vi "find_new_direction.vi"(11 "NXT":T1={"Hardware"="NXT", "Flattened String"=""}) -> (0 "right(T)/left(F)":bool, 1 "angle":dbl, 3 "NXT 2":T1={"Hardware"="NXT", "Flattened String"=""})   [LabVIEW 2012]
uses:
  <vilib>/NXT/Subs/LVHSConnector.ctl
  <vilib>/NXT/Subs/MotorOutput.ctl
  <vilib>/NXT/Block Support/NXT_InputPort.ctl
  <vilib>/NXT/Dual Mode Library/Motors/MotorOn.vi
  <vilib>/NXT/Dual Mode Library/Motors/MotorReverse.vi
  <vilib>/NXT/Dual Mode Library/Motors/MotorBrake.vi
  <vilib>/NXT/Dual Mode Library/Display/clearDisplay.vi
  <vilib>/NXT/Dual Mode Library/Waits/Wait_Num(msec).vi
  <vilib>/NXT/Dual Mode Library/Display/drawLine.vi
  <vilib>/NXT/Dual Mode Library/Waits/Wait_Num.vi
  <vilib>/NXT/Dual Mode Library/Display/drawText.vi
  <vilib>/NXT/Dual Mode Library/Display/drawNumber.vi
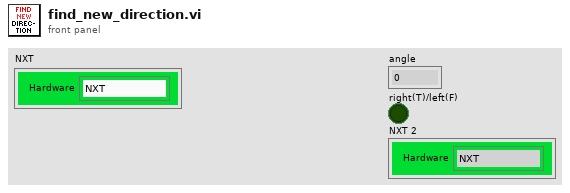
[diagram p1: front panel]
types:
  T1 = typedef "LVHSConnector.ctl" = cluster{"Hardware":string, "Flattened String":string}
  T2 = typedef "MotorOutput.ctl" = u8
  T3 = typedef "NXT_InputPort.ctl" = u8
  T4 = cluster{"x-y*floor(x/y)":i32, "Start X":i16, "x-y*floor(x/y)":i32, i16}
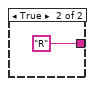
[diagram p6: hidden frame]
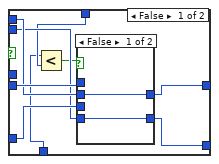
[diagram p9: hidden frame]
diagram:
  w19 = T2 5 items=["Port A"=0, "Port B"=1, "Port C"=2, "Ports A & B"=4, "Ports A & C"=5, "Ports B & C"=6, "All Ports"=3] ("Port (All Ports)")
  w25 = T2 5 items=["Port A"=0, "Port B"=1, "Port C"=2, "Ports A & B"=4, "Ports A & C"=5, "Ports B & C"=6, "All Ports"=3] ("Port (All Ports)")
  w29 = T2 2 items=["Port A"=0, "Port B"=1, "Port C"=2, "Ports A & B"=4, "Ports A & C"=5, "Ports B & C"=6, "as"=3] ("Output Port (All Ports)")
  w27 = T2 0 items=["Port A"=0, "Port B"=1, "Port C"=2, "Ports A & B"=4, "Ports A & C"=5, "Ports B & C"=6, "as"=3] ("Output Port (All Ports)")
  w43 = i16 -1 ("Start X")
  (unwired) FALSE
  w15 = TRUE
  w24 = 35 ("Power (75)")
  # "number of samples"
  # "40"
  # "rotate left"
  # "sweep sensor left"
  # "move sensor back"
  # "if sample angle is > 180, rotate right instead of left"
  # "TODO: pass array length to  find paths"
  # "TODO: pass array size to display array vi"
  # "TODO: pass array length to filter & smooth"
  # "number of distance samples"
  # "degrees"
  # "display chosen location"
  # "display list of areas"
  # "if index > 50;\n  test_index  =  100-index\n\nif current_area <  min_area:\n   if  area > current_area:\n     current_area = area\n     current_index = index\nif current_area >=  min_area:\n\n  if test_index < current_index:\n    current_area = area\n    current_index = index"
  # "morgan stanly analysist internship"
  # "minumum candedata size"
  # "find the closest turn candedate to the forward faceing direction with area over a given minimum\nor the largest if non over the minimum are found"
  # "TODO:  min distance considered, min area"
  # "msecs between distance sampling"
  # "motor power level (for scanning)"
  # "TODO:\n\n combine first and last path condidates (occuring at beginning and end of array-->should be done in the 'find paths' vi\n            \n should have minimum area, take the first one on the left(then right) side that is large enough\n\n     while current_area is less then minimum area:\n            if test_area is greator then current_area:\n                  current_area = test_area\n\ndetermindegress to turn\n\nturn, move forward until some distance is meet (?)"
  # "right max"
  # "left max"
  # "display path candedates"
  # "area"
  # "location"
  # "debug"
  # "screen: 99x63"
  n1 = call <vilib>:"ResetMotor.vi"("NXT"="NXT", "Port (All Ports)"=w25) -> ("NXT"=w26:T1)  [unwired: 2 in]
  n2 = Multiply(x=360.0 ("Max Value"), y=1.45 ("Max Value")) -> (x*y=w20:dbl)
  n3 = call-poly <vilib>:"PolyMotor.vi"("Power (75)"=w24, "NXT"=w26, "Output Port (All Ports)"=w27) -> ("NXT"=w28:T1)  [unwired: 1 in]
  n4 = call-poly <vilib>:"PolyMotor.vi"("Power (75)"=w24, "NXT"=w28, "Output Port (All Ports)"=w29) -> ("NXT"=w23:T1)  [unwired: 1 in]
  n5 = while {
    shift-right: [w78] -> w1
    shift-left: i16[] [] -> [w79]
    tunnel: [w75] -> w18
    tunnel: w15 -> [w74]
    tunnel: 7 -> [w71]
    tunnel: w23 -> [w60]
    tunnel: w20 -> [w57]
    i -> [w72]
    stop <- w58 stop-if-true
    w68 = T2 2 items=["Port A"=0, "Port B"=1, "Port C"=2, "Ports A & B"=4, "Ports A & C"=5, "Ports B & C"=6, "as"=3] ("Output Port (All Ports)")
    w69 = T2 0 items=["Port A"=0, "Port B"=1, "Port C"=2, "Ports A & B"=4, "Ports A & C"=5, "Ports B & C"=6, "as"=3] ("Output Port (All Ports)")
    w80 = T3 3 items=["Port 1", "Port 2", "Port 3", "Port 4"] ("Port (Port 4)")
    n6 = call <vilib>:"Rotation.vi"("NXT"=w60, "Port (Port A)"=w69) -> ("Angle of Rotation"=w67:i32, "NXT"=w70:T1)  [unwired: 1 in]
    n7 = Absolute Value(x=w67) -> (abs(x)=w65:i32)
    n8 = call <vilib>:"Rotation.vi"("NXT"=w70, "Port (Port A)"=w68) -> ("Angle of Rotation"=w66:i32, "NXT"=w59:T1)  [unwired: 1 in]
    n9 = Absolute Value(x=w66) -> (abs(x)=w64:i32)
    n10 = Add(x=w64, y=w65) -> (x+y=w63:i32)
    n11 = Divide(x=w63, y=2) -> (x/y=w61:dbl)
    n12 = Greater Or Equal?(x=w61, y=w57) -> (x >= y?=w58:bool)
    n13 = call <vilib>:"Sonar_cm.vi"("NXT"=w59, "Port (Port 4)"=w80) -> ("Distance (cm)"=w73:i16, "NXT"=w77:T1)  [unwired: 1 in]
    n14 = Build Array (concatenate)(w79, w73) -> (w78:i16[])
    n15 = call-poly <vilib>:"PolyWait.vi"("Time (100 msec)"=w71, "NXT"=w77) -> ("NXT"=w76:T1)  [unwired: 2 in]
    n16 = case shown="True" w74 {
      tunnel: w76 -> [w81 w91]
      tunnel: [w81 w92] -> w75
      tunnel: w73 -> [_ w90]
      tunnel: w72 -> [_ w83]
      frame False {
      }
      frame True {
        n17 = Divide(x=i16 60 ("Start X"), y=i16 255 ("Start X")) -> (x/y=w88:dbl)
        n18 = Multiply(x=w90, y=w88) -> (x*y=w93:dbl)
        n19 = To Word Integer(number=w93) -> (16bit integer=w85:i16)
        n20 = call <vilib>:"quot_Remain.vi"("y"=i16 99 ("Start X"), "x"=w83) -> ("x-y*floor(x/y)"=w84:i32)  [unwired: 1 out]
        n21 = Bundle("x-y*floor(x/y)"=w84, "Start X"=i16 0, "x-y*floor(x/y)"=w84, w85) -> (w86:T4)  [unwired: 1 in]
        n22 = call-poly <vilib>:"PolyDisplay.vi"("Line Parameters"=w86, "NXT"=w91) -> ("NXT"=w92:T1)  [unwired: 2 in]
      }
    }
  }
  n23 = Array Size(array=w1) -> (size(s)=w7:i32)
  n24 = call-poly <vilib>:"PolyMotor.vi"("NXT"=w18, "Port (All Ports)"=w19) -> ("NXT"=w17:T1)  [unwired: 2 in]
  n25 = case shown="True" w15 {
    tunnel: w17 -> [w95 w104]
    tunnel: [w95 w97] -> w16
    tunnel: w1 -> [_ w102]
    frame False {
    }
    frame True {
      # "fit raw data to screen"
      # "pause while displaying raw data"
      n26 = while {
        tunnel: w104 -> [w111]
        tunnel: [w110] -> w100
        stop <- w112 stop-if-true
        n27 = call <vilib>:"readNXTButton.vi"("NXT"=w111) -> ("Yes/No"=w112:bool, "NXT"=w110:T1)  [unwired: 2 in]
      }
      n28 = call-poly <vilib>:"PolyWait.vi"("Time (1 sec)"=i16 1, "NXT"=w100) -> ("NXT"=w99:T1)  [unwired: 2 in]
      n29 = call "radial_array_display.vi"("array"=w102, "clear (T/F)"=TRUE, "NXT"=w99) -> ("NXT 2"=w103:T1)  [unwired: 8 in]
      n30 = while {
        tunnel: w103 -> [w108]
        tunnel: [w107] -> w96
        stop <- w109 stop-if-true
        n31 = call <vilib>:"readNXTButton.vi"("NXT"=w108) -> ("Yes/No"=w109:bool, "NXT"=w107:T1)  [unwired: 2 in]
      }
      n32 = stacked-sequence {
        tunnel: w96 -> [w106]
        tunnel: [w106] -> w97
        frame #0 {
          n33 = Wait (ms)(milliseconds to wait=u32 1000) -> ()  [unwired: 1 out]
        }
      }
    }
  }
  n34 = stacked-sequence {
    tunnel: w1 -> [w117]
    tunnel: [w113] -> w55
    tunnel: w16 -> [w116]
    tunnel: [w116] -> w13
    frame #0 {
      n35 = call "filter_bad_values.vi"("Array 3"=w117) -> ("Array 4"=w114:i32[])  [unwired: 10 in]
      n36 = call "kernal_smooth.vi"("array"=w114) -> ("Array"=w115:i16[])  [unwired: 10 in]
      n37 = call "kernal_smooth.vi"("array"=w115) -> ("Array"=w113:i16[])  [unwired: 10 in]
    }
  }
  n38 = case shown="True" w15 {
    tunnel: w13 -> [w119 w120]
    tunnel: w55 -> [w118 w125]
    tunnel: [w119 w121] -> w52
    tunnel: [w118 w125] -> w54
    frame False {
    }
    frame True {
      # "displaying filtered and smoothed data"
      # "filter and display array"
      n39 = call "radial_array_display.vi"("array"=w125, "NXT"=w120) -> ("NXT 2"=w124:T1)  [unwired: 9 in]
      n40 = while {
        tunnel: w124 -> [w127]
        tunnel: [w126] -> w122
        stop <- w128 stop-if-true
        n41 = call <vilib>:"readNXTButton.vi"("NXT"=w127) -> ("Yes/No"=w128:bool, "NXT"=w126:T1)  [unwired: 2 in]
      }
      n42 = call-poly <vilib>:"PolyWait.vi"("Time (1 sec)"=i16 1, "NXT"=w122) -> ("NXT"=w121:T1)  [unwired: 2 in]
    }
  }
  n43 = call-poly <vilib>:"PolyDisplay.vi"("NXT"=w52) -> ("NXT"=w34:T1)  [unwired: 3 in]
  n44 = stacked-sequence {
    tunnel: w54 -> [w132]
    tunnel: [w131] -> w53
    tunnel: [w130] -> w30
    tunnel: w34 -> [w129]
    tunnel: [w129] -> w33
    frame #0 {
      n45 = call "find_path.vi"("Array"=w132) -> ("debug array"=w131:i32[], "Array 2"=w130:i32[])  [unwired: 9 in]
    }
  }
  n46 = case shown="True" w15 {
    tunnel: w53 -> [w134 w145]
    tunnel: w33 -> [w135 w143]
    tunnel: [w135 w138] -> w48
    tunnel: w54 -> [w133 w146]
    tunnel: [w134 w142] -> _
    tunnel: w7 -> [_ w137]
    tunnel: [w133 w136] -> w9
    frame False {
    }
    frame True {
      n47 = stacked-sequence {
        tunnel: w146 -> [w161]
        tunnel: [w160] -> w136
        tunnel: w145 -> [w151]
        tunnel: w143 -> [w152]
        tunnel: [w152] -> w144
        tunnel: [w151] -> w142
        tunnel: w137 -> [w150]
        frame #0 {
          # "end"
          n48 = Array Size(array=w151) -> (size(s)=w155:i32)
          n49 = Divide(x=w155, y=3) -> (x/y=w153:dbl)
          n50 = for {
            N: w153 -> [_]
            shift-right: [w181] -> _
            shift-left: i16 0 ("Start X") -> [w178]
            shift-right: [w180] -> _
            shift-left: i16 1 ("Start X") -> [w177]
            shift-right: [w169] -> w159
            shift-left: i16[] [] -> [w171]
            tunnel: w151 -> [w176]
            shift-right: [w174] -> w157
            shift-left: i16 0 ("Start X") -> [w175]
            w182 = 3 ("y")
            # "end"
            # "start"
            n51 = Index Array(array=w176, index=w178) -> (element=w173:i32)
            n52 = Subtract(x=w173, y=w175) -> (x-y=w179:i32)
            n53 = for {
              N: w179 -> [_]
              shift-right: [w187] -> w170
              shift-left: w171 -> [w188]
              n54 = Build Array (concatenate)(w188, i16 0 ("Start X")) -> (w187:i16[])
            }
            n55 = Index Array(array=w176, index=w177) -> (element=w174:i32)
            n56 = Subtract(x=w174, y=w173) -> (x-y=w172:i32)
            n57 = for {
              N: w172 -> [_]
              shift-right: [w183] -> w169
              shift-left: w170 -> [w184]
              n58 = Build Array (concatenate)(w184, i16 1 ("Start X")) -> (w183:i16[])
            }
            n59 = Add(x=w178, y=w182) -> (x+y=w181:i32)
            n60 = Add(x=w177, y=w182) -> (x+y=w180:i32)
          }
          n61 = Subtract(x=w150, y=w157) -> (x-y=w156:i32)
          n62 = for {
            N: w156 -> [_]
            shift-right: [w167] -> w158
            shift-left: w159 -> [w168]
            n63 = Build Array (concatenate)(w168, i16 0 ("Start X")) -> (w167:i16[])
          }
          n64 = Multiply(x=w158, y=w161) -> (x*y=w160:i16[])
        }
      }
      n65 = call "radial_array_display.vi"("array"=w136, "NXT"=w144) -> ("NXT 2"=w141:T1)  [unwired: 9 in]
      n66 = while {
        tunnel: w141 -> [w148]
        tunnel: [w147] -> w139
        stop <- w149 stop-if-true
        n67 = call <vilib>:"readNXTButton.vi"("NXT"=w148) -> ("Yes/No"=w149:bool, "NXT"=w147:T1)  [unwired: 2 in]
      }
      n68 = call-poly <vilib>:"PolyWait.vi"("Time (1 sec)"=sgl 2.0, "NXT"=w139) -> ("NXT"=w138:T1)  [unwired: 2 in]
    }
  }
  n69 = case shown="True" w15 {
    tunnel: w48 -> [w189 w200]
    tunnel: w30 -> [_ w194]
    tunnel: [w189 w190] -> w46
    frame False {
    }
    frame True {
      # "display list of areas"
      # "0 for list of positions"
      n70 = Array Size(array=w194) -> (size(s)=w198:i32)
      n71 = Divide(x=w198, y=2) -> (x/y=w196:dbl)
      n72 = To Word Integer(number=w196) -> (16bit integer=w195:i16)
      n73 = for {
        N: w195 -> [_]
        tunnel: w200 -> [w213]
        tunnel: [w213] -> w202
        shift-right: [w214] -> w201
        shift-left: "" ("Text") -> [w216]
        shift-right: [w211] -> _
        shift-left: i16 1 ("Start X") -> [w209]
        tunnel: w194 -> [w208]
        n74 = Index Array(array=w208, index=w209) -> (element=w207:i32)
        n75 = call <vilib>:"NXT_floatToString.vi"("number"=w207) -> ("string"=w215:string)
        n76 = Concatenate Strings(w216, " " ("Text"), w215) -> (w214:string)
        n77 = Add(x=w209, y=i16 2 ("Start X")) -> (x+y=w211:i16)
      }
      n78 = call-poly <vilib>:"PolyDisplay.vi"("Text"=w201, "NXT"=w202) -> ("NXT"=w193:T1)  [unwired: 2 in]
      n79 = while {
        tunnel: w193 -> [w205]
        tunnel: [w204] -> w191
        stop <- w206 stop-if-true
        n80 = call <vilib>:"readNXTButton.vi"("NXT"=w205) -> ("Yes/No"=w206:bool, "NXT"=w204:T1)  [unwired: 2 in]
      }
      n81 = call-poly <vilib>:"PolyWait.vi"("Time (1 sec)"=i16 1, "NXT"=w191) -> ("NXT"=w190:T1)  [unwired: 2 in]
    }
  }
  n82 = Array Size(array=w30) -> (size(s)=w31:i32)
  n83 = Divide(x=w31, y=i16 2 ("Start X")) -> (x/y=w49:dbl)
  n84 = To Byte Integer(number=w49) -> (8bit integer=w47:i8)
  n85 = for {
    N: w47 -> [_]
    tunnel: w30 -> [w238]
    shift-right: [w237] -> _
    shift-left: i16 0 ("Start X") -> [w220]
    shift-right: [w236] -> _
    shift-left: i16 1 ("Start X") -> [w234]
    shift-right: [w229] -> w6
    shift-left: w43 -> [w224]
    shift-right: [w228] -> w42
    shift-left: w43 -> [w221]
    tunnel: w46 -> [w233]
    tunnel: i16 700 ("Start X") -> [w222]
    tunnel: [w233] -> w40
    tunnel: w7 -> [w218]
    w235 = i16 2 ("Start X")
    # "area"
    # "position"
    n86 = Divide(x=w218, y=i16 2 ("Start X")) -> (x/y=w217:dbl)
    n87 = Index Array(array=w238, index=w234) -> (element=w230:i32)
    n88 = Index Array(array=w238, index=w220) -> (element=w223:i32)
    n89 = Less?(x=w221, y=w222) -> (x < y?=w231:bool)
    n90 = Greater Or Equal?(x=w224, y=w217) -> (x >= y?=w232:bool)
    n91 = Greater Or Equal?(x=w223, y=w217) -> (x >= y?=w226:bool)
    n92 = case shown="True" w232 {
      tunnel: w224 -> [w268 w270]
      tunnel: [w268 w271] -> w227
      tunnel: w218 -> [_ w269]
      frame False {
      }
      frame True {
        n93 = Subtract(x=w269, y=w270) -> (x-y=w271:i32)
      }
    }
    n94 = case shown="True" w226 {
      tunnel: w223 -> [w239 w242]
      tunnel: [w239 w241] -> w225
      tunnel: w218 -> [_ w240]
      frame False {
      }
      frame True {
        n95 = Subtract(x=w240, y=w242) -> (x-y=w241:i32)
      }
    }
    n96 = case shown="True" w231 {
      tunnel: w223 -> [w251 w261]
      tunnel: w230 -> [w250 w259]
      tunnel: [w249 w260] -> w229
      tunnel: [w248 w258] -> w228
      tunnel: w227 -> [w245 _]
      tunnel: w225 -> [w244 _]
      tunnel: w224 -> [w247 w257]
      tunnel: w221 -> [w246 w256]
      tunnel: w221 -> [_ w263]
      frame False {
        n97 = Less?(x=w244, y=w245) -> (x < y?=w243:bool)
        n98 = case shown="False" w243 {
          tunnel: w251 -> [_ w255]
          tunnel: w250 -> [_ w254]
          tunnel: [w253 w255] -> w249
          tunnel: [w252 w254] -> w248
          tunnel: w247 -> [w253 _]
          tunnel: w246 -> [w252 _]
          frame False {
          }
          frame True {
          }
        }
      }
      frame True {
        n99 = Greater?(x=w259, y=w263) -> (0:w262:bool)
        n100 = case shown="True" w262 {
          tunnel: w261 -> [_ w267]
          tunnel: [w264 w267] -> w260
          tunnel: w259 -> [_ w266]
          tunnel: [w265 w266] -> w258
          tunnel: w257 -> [w264 _]
          tunnel: w256 -> [w265 _]
          frame False {
          }
          frame True {
          }
        }
      }
    }
    n101 = Add(x=w220, y=w235) -> (x+y=w237:i16)
    n102 = Add(x=w234, y=w235) -> (x+y=w236:i16)
  }
  n103 = Divide(x=w6, y=w7) -> (x/y=w5:dbl)
  n104 = Divide(x=w7, y=i16 2 ("Start X")) -> (x/y=w35:dbl)
  n105 = Greater Or Equal?(x=w6, y=w35) -> (x >= y?=w39:bool)
  n106 = case shown="True" w39 {
    tunnel: w6 -> [w272 w274]
    tunnel: [w272 w273] -> w38
    tunnel: w7 -> [_ w275]
    frame False {
    }
    frame True {
      n107 = Subtract(x=w275, y=w274) -> (x-y=w273:i32)
    }
  }
  n108 = Multiply(x=6.283185307179586 ("Pi Multiplied By 2"), y=w5) -> (x*y=w4:dbl)
  n109 = Add(x=1.5707963267948966 ("Pi Divided By 2"), y=w4) -> (x+y=w2:dbl)
  n110 = Divide(x=w38, y=w7) -> (x/y=w11:dbl)
  n111 = Greater Or Equal?(x=w6, y=w35) -> (x >= y?=w8:bool)
  "right(T)/left(F)" <- w8
  n112 = Multiply(x=i16 360 ("Start X"), y=w11) -> (x*y=w10:dbl)
  "angle" <- w10
  n113 = case shown="True" w15 {
    tunnel: w40 -> [w276 w278]
    tunnel: [w276 w302] -> w37
    tunnel: w42 -> [_ _]
    tunnel: w2 -> [_ w297]
    tunnel: w10 -> [_ w298]
    tunnel: w9 -> [_ w282]
    tunnel: w8 -> [_ w281]
    frame False {
      # "turn right"
    }
    frame True {
      w294 = i16 100 ("Start X")
      w299 = i16 2 items=["1", "2", "3", "4", "5", "6", "7", "8"] ("Line")
      w301 = i16 1 items=["1", "2", "3", "4", "5", "6", "7", "8"] ("Line")
      w291 = i16 49 ("Start X")
      w290 = i16 31 ("Start X")
      # "dont erase"
      # "turn left"
      n114 = call <vilib>:"cosine.vi"("x"=w297) -> ("cos(x)"=w296:sgl)
      n115 = call <vilib>:"sine.vi"("x"=w297) -> ("sin(x)"=w295:sgl)
      n116 = call-poly <vilib>:"PolyDisplay.vi"("NXT"=w278) -> ("NXT"=w277:T1)  [unwired: 3 in]
      n117 = Multiply(x=w294, y=w295) -> (x*y=w292:sgl)
      n118 = Multiply(x=w294, y=w296) -> (x*y=w293:sgl)
      n119 = Add(x=w292, y=w290) -> (x+y=w286:sgl)
      n120 = Add(x=w291, y=w293) -> (x+y=w287:sgl)
      n121 = call-poly <vilib>:"PolyDisplay.vi"("number"=w298, "NXT"=w277, "Line"=w301) -> ("NXT"=w305:T1)  [unwired: 1 in]
      n122 = To Word Integer(number=w286) -> (16bit integer=w288:i16)
      n123 = To Word Integer(number=w287) -> (16bit integer=w289:i16)
      n124 = Bundle("Start X"=w291, "Start X"=w290, w289, w288) -> (w285:cluster{"Start X":i16, "Start X":i16, i16, i16})  [unwired: 1 in]
      n125 = case shown="False" w281 {
        tunnel: ["L" "R"] -> w280
        frame False {
        }
        frame True {
        }
      }
      n126 = call-poly <vilib>:"PolyDisplay.vi"("Text"=w280, "NXT"=w305, "Line"=w299) -> ("NXT"=w284:T1)  [unwired: 1 in]
      n127 = call "radial_array_display.vi"("array"=w282, "clear (T/F)"=FALSE, "NXT"=w284) -> ("NXT 2"=w283:T1)  [unwired: 8 in]
      n128 = call-poly <vilib>:"PolyDisplay.vi"("Line Parameters"=w285, "NXT"=w283) -> ("NXT"=w300:T1)  [unwired: 2 in]
      n129 = while {
        tunnel: w300 -> [w309]
        tunnel: [w308] -> w303
        stop <- w310 stop-if-true
        n130 = call <vilib>:"readNXTButton.vi"("NXT"=w309) -> ("Yes/No"=w310:bool, "NXT"=w308:T1)  [unwired: 2 in]
      }
      n131 = call-poly <vilib>:"PolyWait.vi"("Time (1 sec)"=i16 1, "NXT"=w303) -> ("NXT"=w302:T1)  [unwired: 2 in]
    }
  }
  "NXT 2" <- w37
